vi "GET.comics.month.vi"(4 "series offset":u32, 5 "request specific headers":T2[](array[typedef]), 6 "Number of Series to GET":u32, 7 "timeout (60000)":i32=60000, 8 "error in (no error)":errorcluster, 11 "REST Client in":refnum<class "REST Client.lvclass">) -> (0 "error out":errorcluster, 2 "data":T1, 3 "REST Client out":refnum<class "REST Client.lvclass">)   [LabVIEW 2024]
uses:
  <vilib>/addons/_JKI.lib/REST Client/classes/REST Client/HTTP Header.ctl
  <vilib>/NI/Advanced HTTP Client/Header--Combo Box.ctl
  <vilib>/addons/_JKI.lib/REST Client/classes/REST Client/REST Client.lvclass
  TypeDefs/comics.reply--cluster.ctl
  <vilib>/NI/Advanced HTTP Client/Session.lvclass
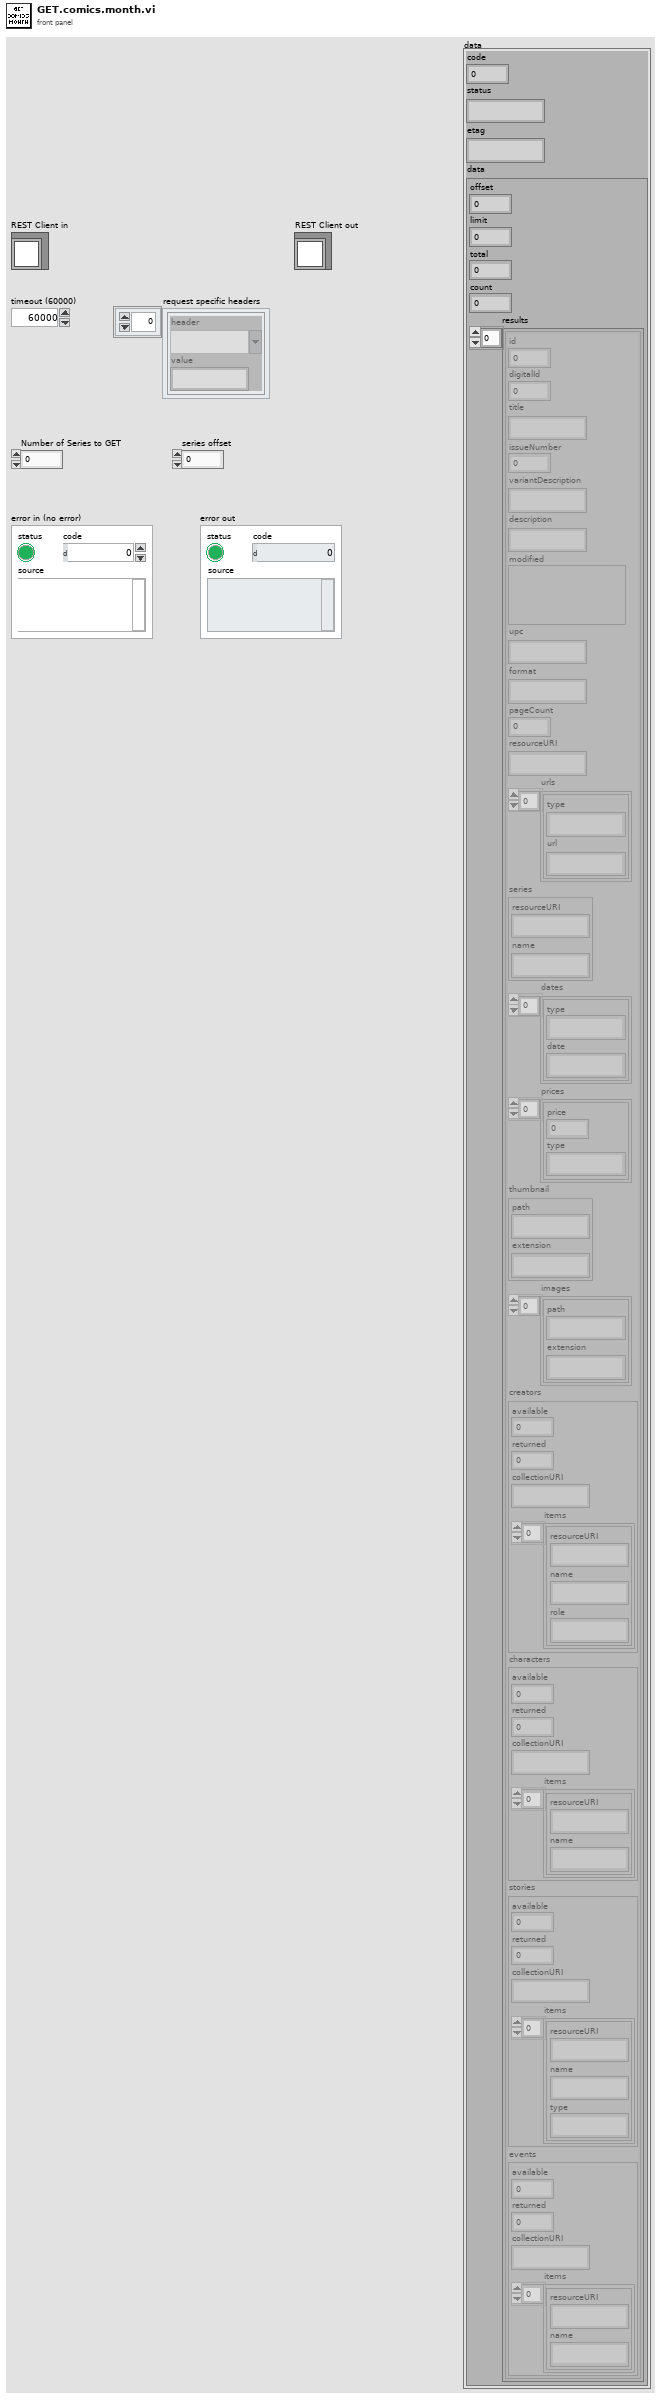
[diagram p1: front panel]
types:
  T1 = typedef "comics.reply--cluster.ctl" = cluster{"code":i32, "status":string, "etag":string, "data":cluster{"offset":i32, "limit":i32, "total":i32, "count":i32, "results":cluster{"id":i32, "digitalId":i32, "title":string, "issueNumber":i32, "variantDescription":string, "description":string, "modified":variant, "upc":string, "format":string, "pageCount":i32, "resourceURI":string, "urls":cluster{"type":string, "url":string}[], "series":cluster{"resourceURI":string, "name":string}, "dates":cluster{"type":string, "date":string}[], "prices":cluster{"price":dbl, "type":string}[], "thumbnail":cluster{"path":string, "extension":string}, "images":cluster{"path":string, "extension":string}[], "creators":cluster{"available":i32, "returned":i32, "collectionURI":string, "items":cluster{"resourceURI":string, "name":string, "role":string}[]}, "characters":cluster{"available":i32, "returned":i32, "collectionURI":string, "items":cluster{"resourceURI":string, "name":string}[]}, "stories":cluster{"available":i32, "returned":i32, "collectionURI":string, "items":cluster{"resourceURI":string, "name":string, "type":string}[]}, "events":cluster{"available":i32, "returned":i32, "collectionURI":string, "items":cluster{"resourceURI":string, "name":string}[]}}[]}}
  T2 = typedef "REST Client.lvlib/REST Client.lvclass/HTTP Header.ctl" = cluster{"header":T3, "value":string}
  T3 = typedef "lib_NI_Advanced HTTP Client.lvlib/Session.lvclass/Header--Combo Box.ctl" = string
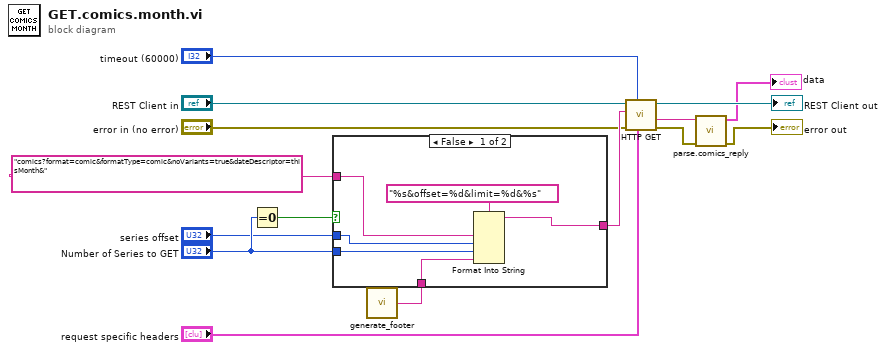
[diagram p0: block diagram]
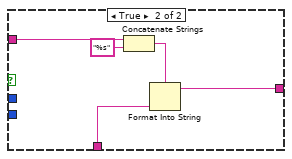
[diagram p2: hidden frame]
diagram:
  n1 = Equal To 0?(x="Number of Series to GET") -> (x = 0?=w3:bool)
  n2 = call "generate_footer.vi"() -> ("footer"=w10:string)  [unwired: 1 in]
  n3 = case shown="False" w3 {
    tunnel: [w21 w26] -> w11
    tunnel: w10 -> [w20 w25]
    tunnel: "series offset" -> [w19 _]
    tunnel: "Number of Series to GET" -> [w18 _]
    tunnel: "comics?format=comic&formatType=comic&noVariants=true&dateDescriptor=thisMonth&" ("Path") -> [w16 w24]
    frame False {
      n4 = Format Into String(format string="%s&offset=%d&limit=%d&%s" ("Path"), w16, w19, w18, w20) -> (resulting string=w21:string)  [unwired: 2 in, 1 out]
    }
    frame True {
      n5 = Concatenate Strings(w24, "%s" ("string")) -> (w23:string)
      n6 = Format Into String(format string=w23, w25) -> (resulting string=w26:string)  [unwired: 2 in, 1 out]
    }
  }
  n7 = call-dynamic "HTTP GET.vi"("request specific headers"="request specific headers", "timeout (0 = Use Default)"="timeout (60000)", "error in (no error)"="error in (no error)", "Path"=w11, "REST Client in"="REST Client in") -> ("error out"=w13:errorcluster, "Response body"=w12:string, "REST Client out"=→"REST Client out":refnum<class "REST Client.lvclass">)  [unwired: 1 in, 3 out]
  n8 = call "parse.comics_reply.vi"("error in"=w13, "string in"=w12) -> ("error out"=→"error out":errorcluster, "data"=→"data":T1)  [unwired: 8 in]
